vi "Find Variable Using Monkey Job Result.vi"(1 "Monkeys":T1, 2 "Variable":string, 3 "Monkey":string, 4 "Job Result":u64) -> (0 "Variable Value":u64)   [LabVIEW 2020, in "AoC 2022.lvlib"]
uses:
  AoC 2022.lvlib
  Day 11 - Monkey in the Middle/private/Monkeys.ctl
  Day 11 - Monkey in the Middle/private/Monkey.ctl
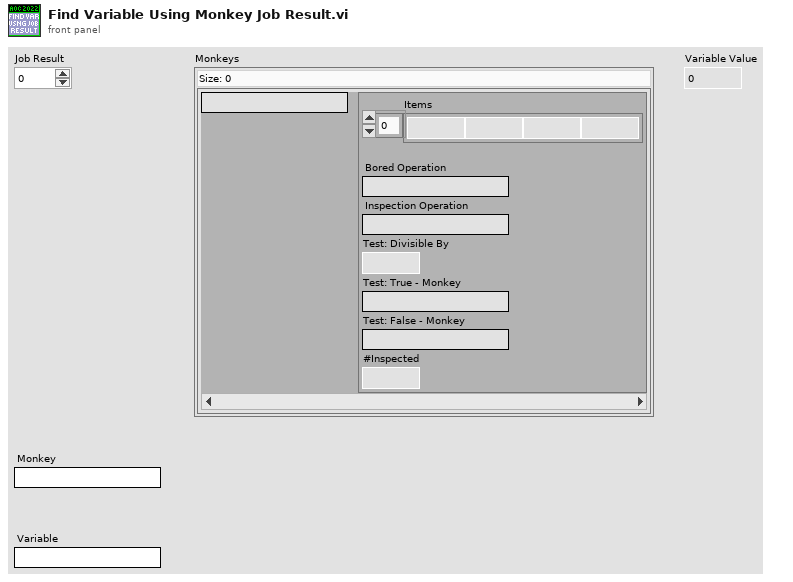
[diagram p1: front panel]
types:
  T1 = typedef "AoC 2022.lvlib/Monkeys.ctl" = map{string, T2}
  T2 = typedef "AoC 2022.lvlib/Monkey.ctl" = cluster{"Items":u64[], "Bored Operation":string, "Inspection Operation":string, "Test: Divisible By":u64, "Test: True - Monkey":string, "Test: False - Monkey":string, "#Inspected":i32}
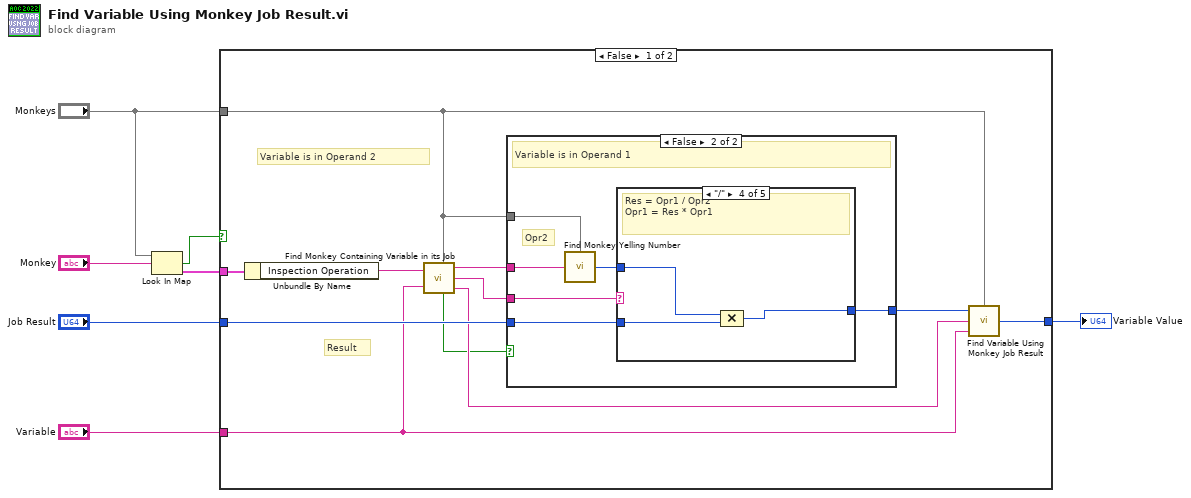
[diagram p0: block diagram]
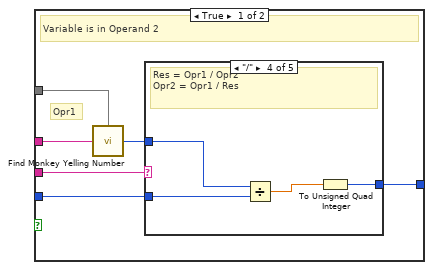
[diagram p2: hidden frame]
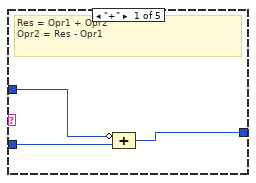
[diagram p3: hidden frame]
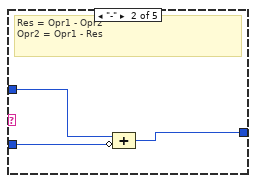
[diagram p4: hidden frame]
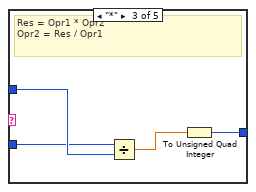
[diagram p5: hidden frame]
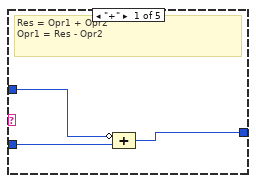
[diagram p7: hidden frame]
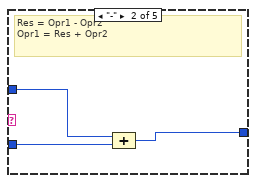
[diagram p8: hidden frame]
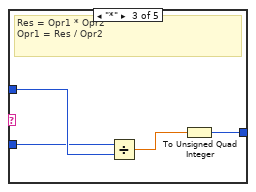
[diagram p9: hidden frame]
diagram:
  n1 = Look In Map(map="Monkeys", key="Monkey") -> (key not found?=w1:bool, value=w6:T2)  [unwired: 1 in]
  n2 = case shown="False" w1 {
    tunnel: w6 -> [w18 _]
    tunnel: "Job Result" -> [w14 w60]
    tunnel: "Monkeys" -> [w10 _]
    tunnel: "Variable" -> [w12 _]
    tunnel: [w11 w60] -> w2
    frame False {
      # "Variable is in Operand 2"
      # "Result"
      n3 = Unbundle By Name(w18) -> ("Inspection Operation"=w17:string)
      n4 = call "Find Monkey Containing Variable in its Job.vi"("Monkeys"=w10, "Variable"=w12, "Monkey Job Statement"=w17) -> ("Monkey having Variable in its Job"=w13:string, "Variable is in Right Monkey's Job ?"=w9:bool, "Operator"=w15:string, "Monkey not having Variable in its Job"=w16:string)
      n5 = case shown="False" w9 {
        tunnel: w16 -> [w24 w45]
        tunnel: w15 -> [w22 w43]
        tunnel: w14 -> [w21 w42]
        tunnel: w10 -> [w23 w44]
        tunnel: [w19 w40] -> w8
        frame True {
          # "Opr1"
          # "Variable is in Operand 2"
          n6 = call "Find Monkey Yelling Number.vi"("Monkey"=w24, "Monkeys"=w23) -> ("Monkey Yelling Number"=w20:u64)
          n7 = case shown="\"/\"" w22 {
            tunnel: w21 -> [w26 w29 w33 w37 w39]
            tunnel: w20 -> [w27 w30 w34 w38 _]
            tunnel: [w25 w28 w31 w35 w39] -> w19
            frame "+" {
              # "Res = Opr1 + Opr2\nOpr2 = Res - Opr1"
              n8 = Compound Arithmetic op=ADD(invert w27, w26) -> (w25:u64)
            }
            frame "-" {
              # "Res = Opr1 - Opr2\nOpr2 = Opr1 - Res"
              n9 = Compound Arithmetic op=ADD(w30, invert w29) -> (w28:u64)
            }
            frame "*" {
              # "Res = Opr1 * Opr2\nOpr2 = Res / Opr1"
              n10 = Divide(x=w33, y=w34) -> (x/y=w32:dbl)
              n11 = To Unsigned Quad Integer(1:w32) -> (0:w31:u64)
            }
            frame "/" {
              # "Res = Opr1 / Opr2\nOpr2 = Opr1 / Res"
              n12 = Divide(x=w38, y=w37) -> (x/y=w36:dbl)
              n13 = To Unsigned Quad Integer(1:w36) -> (0:w35:u64)
            }
            frame Default {
            }
          }
        }
        frame False {
          # "Opr2"
          # "Variable is in Operand 1"
          n14 = call "Find Monkey Yelling Number.vi"("Monkey"=w45, "Monkeys"=w44) -> ("Monkey Yelling Number"=w41:u64)
          n15 = case shown="\"/\"" w43 {
            tunnel: w42 -> [w47 w50 w54 w57 w59]
            tunnel: w41 -> [w48 w51 w55 w58 _]
            tunnel: [w46 w49 w52 w56 w59] -> w40
            frame "+" {
              # "Res = Opr1 + Opr2\nOpr1 = Res - Opr2"
              n16 = Compound Arithmetic op=ADD(invert w48, w47) -> (w46:u64)
            }
            frame "-" {
              # "Res = Opr1 - Opr2\nOpr1 = Res + Opr2"
              n17 = Compound Arithmetic op=ADD(w51, w50) -> (w49:u64)
            }
            frame "*" {
              # "Res = Opr1 * Opr2\nOpr1 = Res / Opr2"
              n18 = Divide(x=w54, y=w55) -> (x/y=w53:dbl)
              n19 = To Unsigned Quad Integer(1:w53) -> (0:w52:u64)
            }
            frame "/" {
              # "Res = Opr1 / Opr2\nOpr1 = Res * Opr1"
              n20 = Compound Arithmetic op=MULTIPLY(w58, w57) -> (w56:u64)
            }
            frame Default {
            }
          }
        }
      }
      n21 = call "Find Variable Using Monkey Job Result.vi"("Monkeys"=w10, "Variable"=w12, "Monkey"=w13, "Job Result"=w8) -> ("Variable Value"=w11:u64)
    }
    frame True {
    }
  }
  "Variable Value" <- w2
